vi "Get I Am.vi"(8 "error in (no error)":errorcluster, 11 "niDTS WLAN DUT in":refnum<class "niDTS WLAN Dut.lvclass">) -> (0 "error out":errorcluster, 2 "I Am":string, 3 "niDTS WLAN DUT out":refnum<class "niDTS WLAN Dut.lvclass">)   [LabVIEW 2015, in "niDTS WLAN.lvlib" / "niDTS WLAN Dut.lvclass"]
uses:
  niDTS WLAN Dut.lvclass
panel:
  # "This is used for testing the dispatching of the plugins"
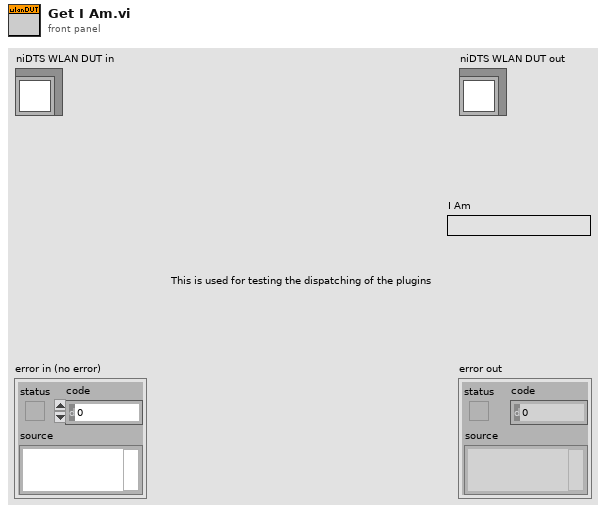
[diagram p1: front panel]
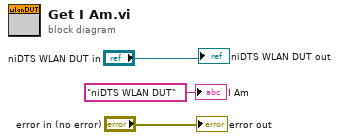
[diagram p0: block diagram]
diagram:
  "error out" <- "error in (no error)"
  "niDTS WLAN DUT out" <- "niDTS WLAN DUT in"
  "I Am" <- "niDTS WLAN DUT" ("I Am")
